vi "FloatToDaData.vi"(2 "代表下限":dbl, 3 "代表上线":dbl, 4 "数值输入控件":dbl) -> (0 "x与y?-低位":u32 format="%x", 1 "floor(x/y)-高位":i16 format="%x")   [LabVIEW 2014]
panel:
  out "输出变量 4":dbl
  out "输出变量 3":u32 format="%x"
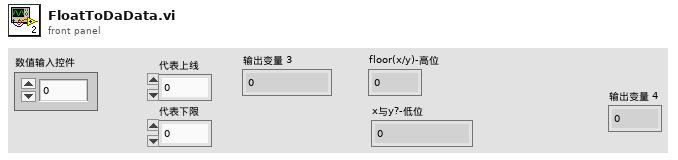
[diagram p1: front panel]
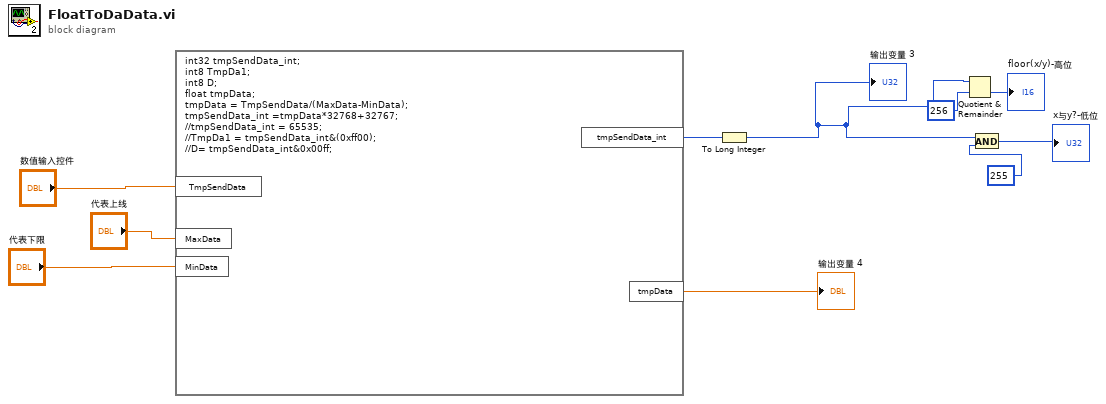
[diagram p0: block diagram]
diagram:
  n1 = formula code="int32 tmpSendData_int;\nint8 TmpDa1;\nint8 D;\nfloat tmpData;\ntmpData = TmpSendData/(MaxData-MinData);\ntmpSendData_int =tmpData*32768+32767;\t\n//tmpSendData_int = 65535;\n//TmpDa1 = tmpSendData_int&(0xff00);\n//D= tmpSendData_int&0x00ff;"("MaxData"="代表上线", "MinData"="代表下限", "TmpSendData"="数值输入控件") -> ("tmpSendData_int"=w2:i32, "tmpData"=→"输出变量 4":dbl)
  n2 = To Long Integer(number=w2) -> (32bit integer=w1:i32)
  "输出变量 3" <- w1
  n3 = Quotient & Remainder(x=w1, y=i16 256) -> (floor(x/y)=→"floor(x/y)-高位":i32)  [unwired: 1 out]
  n4 = And(x=w1, y=i16 255) -> (x .and. y?=→"x与y?-低位":i32)
